vi "Emulate_ELYSE_Clock.vi"   [LabVIEW 2020, in "DAQmxTaksContainer_General.lvclass"]
uses:
  DAQmxTaksContainer_General.lvclass
  dependecies/globalVarII.vi
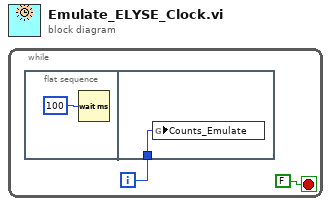
[diagram p0: block diagram]
diagram:
  n1 = while {
    i -> [w1]
    stop <- FALSE stop-if-true
    n2 = flat-sequence {
      tunnel: w1 -> [w4]
      frame #0 {
        n3 = Wait (ms)(milliseconds to wait=u32 100) -> ()  [unwired: 1 out]
      }
      frame #1 {
        n4 = global write "globalVarII.vi" "Counts_Emulate"(w4) -> ()
      }
    }
  }
